vi "Format Array to String.vi"(1 "Input Array":string[][](array[string])) -> (0 "String Out":string)   [LabVIEW 2013]
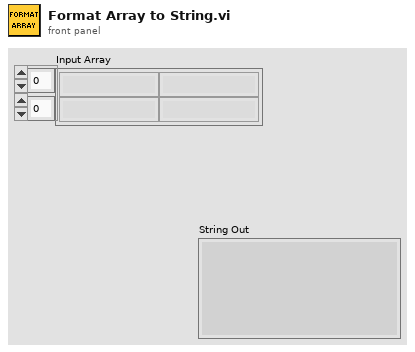
[diagram p1: front panel]
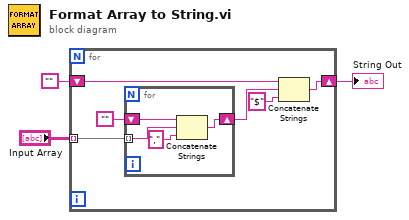
[diagram p0: block diagram]
diagram:
  n1 = for {
    tunnel: "Input Array" -> [w9] mode=indexing
    shift-right: [w6] -> w2
    shift-left: "" -> [w5]
    n2 = for {
      tunnel: w9 -> [w10] mode=indexing
      shift-right: [w13] -> w8
      shift-left: "" -> [w12]
      n3 = Concatenate Strings(w12, w10, "," ("string")) -> (w13:string)
    }
    n4 = Concatenate Strings(w5, w8, "$" ("string")) -> (w6:string)
  }
  "String Out" <- w2
